vi "FTW-JSON-Format-Boolean.vi"(1 "LabVIEW Boolean":bool) -> (0 "JSON Boolean":string)   [LabVIEW 2012]
panel:
  # "Inputs"
  # "Outputs"
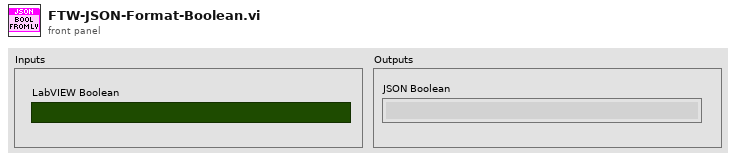
[diagram p1: front panel]
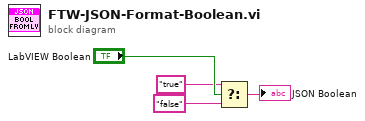
[diagram p0: block diagram]
diagram:
  n1 = Select(t="true", s="LabVIEW Boolean", f="false") -> (s? t:f=→"JSON Boolean":string)
